vi "ex1_digital.vi"() -> ()   [LabVIEW 2018]
panel:
  out "Boolean 2":bool
  in  "Boolean":bool
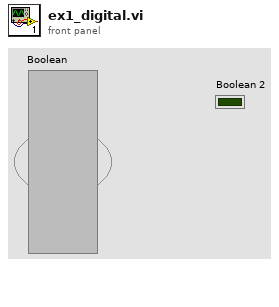
[diagram p1: front panel]
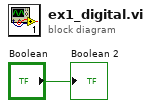
[diagram p0: block diagram]
diagram:
  "Boolean 2" <- "Boolean"
